vi "basicArray.vi"() -> ()   [LabVIEW 2021]
panel:
  out "Col 0":dbl[](array[numeric])
  out "Row 0":dbl[](array[numeric])
  out "element 3":dbl
  in  "index (col)":i32
  in  "index (row)":i32
  out "Numeric Array 3 Size 2":i32[](array[numeric])
  in  "Numeric Array 4":dbl[][](array[numeric])
  out "element 2":i32
  in  "index":i32
  out "Array Size Is":i32[](array[numeric])
  out "initialized array":dbl[][](array[numeric])
  in  "element":dbl
  out "Array Constant Size":i32
  out "Numeric Array 3 Size":i32[](array[numeric])
  out "Numeric Array Size":i32
  in  "Numeric Array 3":dbl[][](array[numeric])
  in  "Bool Array":bool[](array[boolean])
  in  "String Array":string[](array[string])
  in  "Numeric Array":dbl[](array[numeric])
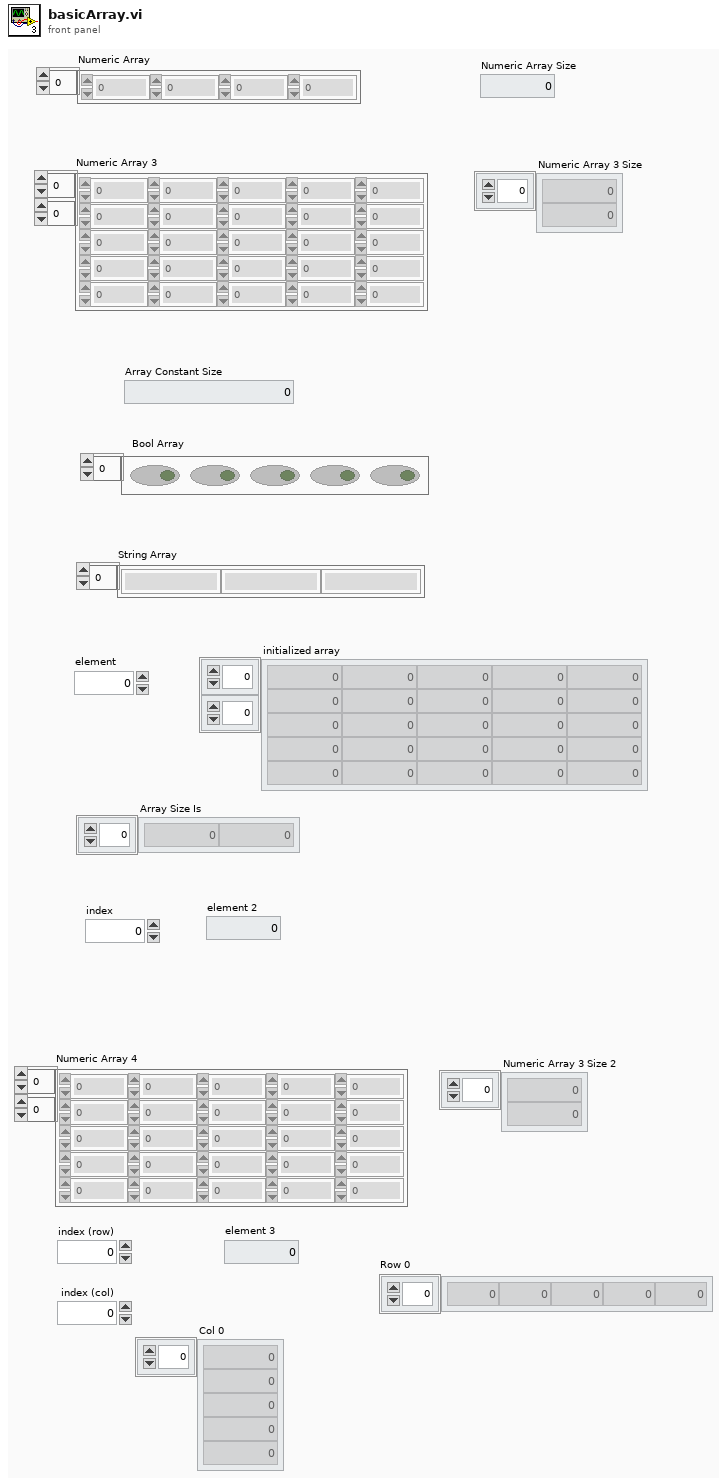
[diagram p1: front panel]
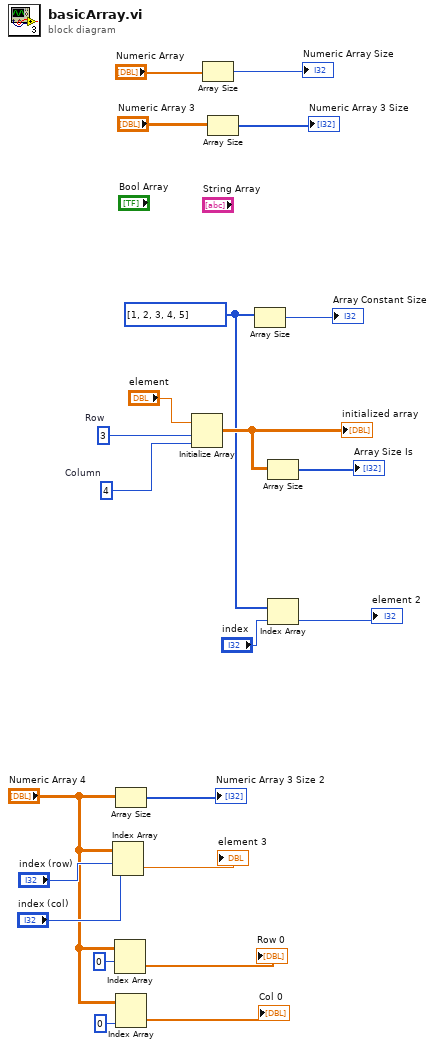
[diagram p0: block diagram]
diagram:
  w15 = 4  # Column
  w16 = 3  # Row
  w12 = i32[] [1, 2, 3, 4, 5]
  n1 = Index Array(array="Numeric Array 4", index (row)="index (row)", index (col)="index (col)") -> (element=→"element 3":dbl)
  n2 = Index Array(array="Numeric Array 4", index (row)=0) -> (element=→"Row 0":dbl[])  [unwired: 1 in]
  n3 = Array Size(array="Numeric Array 4") -> (size(s)=→"Numeric Array 3 Size 2":i32[])
  n4 = Index Array(array="Numeric Array 4", index (col)=0 ("disabled index (col)")) -> (element=→"Col 0":dbl[])  [unwired: 1 in]
  n5 = Initialize Array "Initialize Array"("element", w16, w15) -> (w14:dbl[][])
  "initialized array" <- w14
  n6 = Array Size(array="Numeric Array") -> (size(s)=→"Numeric Array Size":i32)
  n7 = Array Size(array="Numeric Array 3") -> (size(s)=→"Numeric Array 3 Size":i32[])
  n8 = Array Size(array=w12) -> (size(s)=→"Array Constant Size":i32)
  n9 = Array Size(array=w14) -> (size(s)=→"Array Size Is":i32[])
  n10 = Index Array(array=w12, index="index") -> (element=→"element 2":i32)
